vi "Baseband Transmission-Formula.vi"() -> ()   [LabVIEW 2013]
uses:
  <vilib>/Analysis/2dsp.llb/1D Convolution (DBL).vi
  <vilib>/Analysis/2dsp.llb/Decimate (single shot, DBL).vi
  <vilib>/Analysis/2dsp.llb/Upsample (DBL).vi
  <vilib>/Analysis/NI_AALBase.lvlib
  <vilib>/Analysis/NI_AALPro.lvlib
panel:
  in  "alpha":dbl
  in  "Sinc Samples":i32=65
  out "Recovered Bits":i32[](array[numeric])
  in  "stop":bool
  in  "UpSample Factor":i32(slide)=74 scale=1.0..100.0
  out "Symbol":dbl[](array[numeric])
  in  "Bit":i32[](array[numeric])=[0, 0, 0, 1, 0, 1, 1, 1, 0, 0]
  in  "Pulse Shaping Function":enum16{"Sinc ", "Rcosine"}(ring)=enum."Rcosine"
  out "Pulse Shaping":dbl[][](graph)
  out "Baseband":dbl[](graph)
  # "Baseband Transmission"
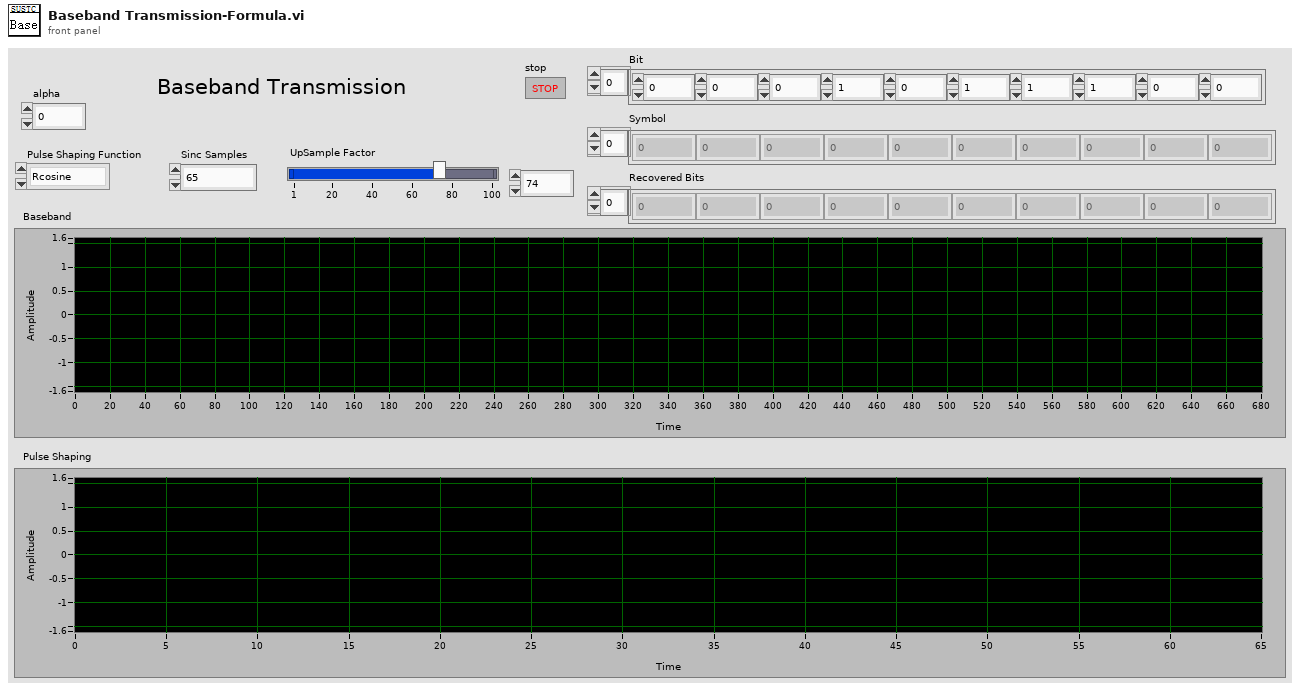
[diagram p1: front panel]
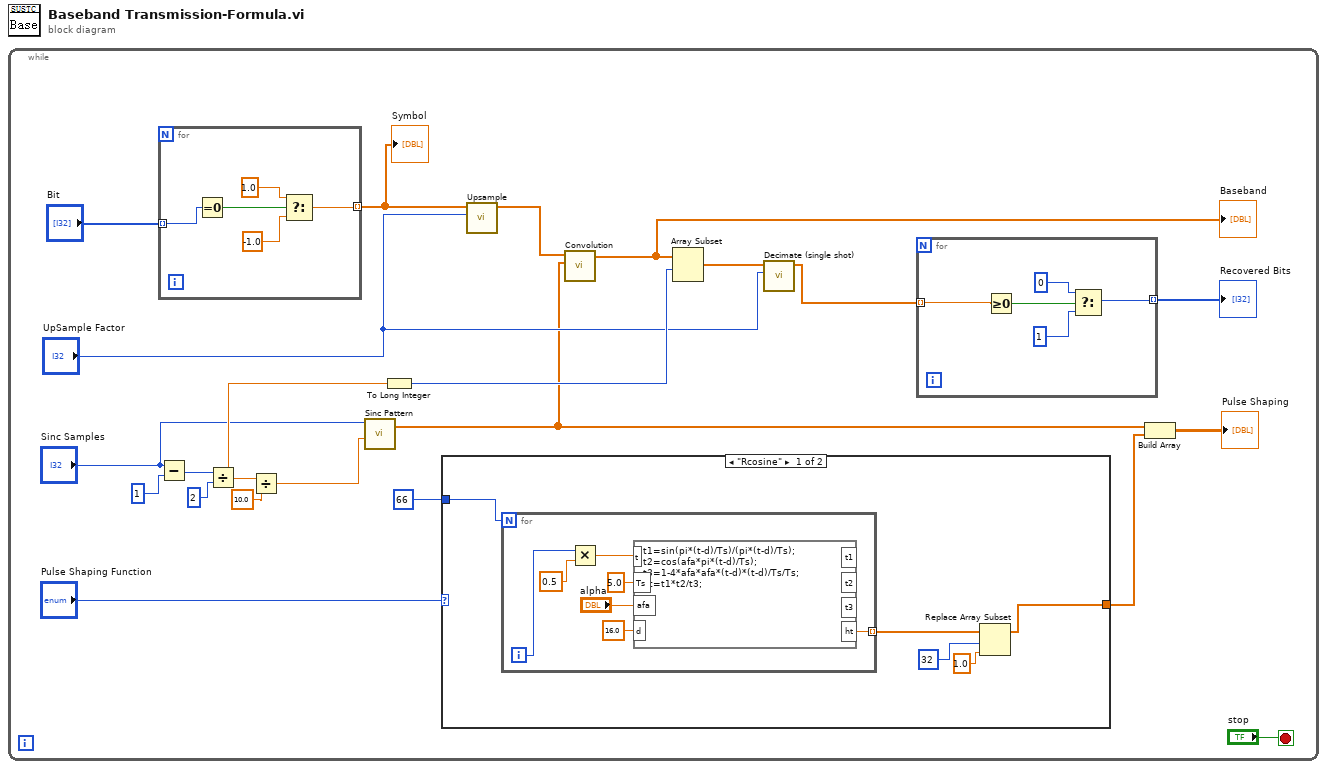
[diagram p0: block diagram]
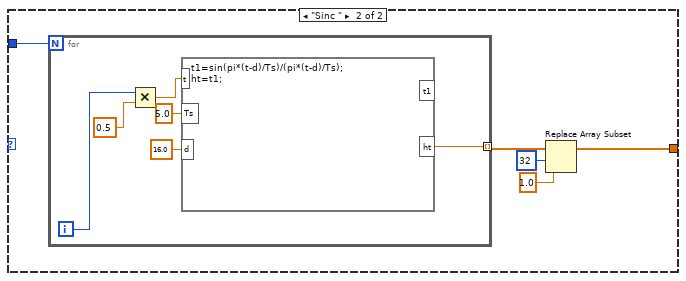
[diagram p2: hidden frame]
diagram:
  n1 = while {
    stop <- "stop" stop-if-true
    n2 = for {
      tunnel: [w52] -> w11 mode=indexing
      tunnel: "Bit" -> [w51] mode=indexing
      n3 = Equal To 0?(x=w51) -> (x = 0?=w55:bool)
      n4 = Select(t=1.0, s=w55, f=-1.0) -> (s? t:f=w52:dbl)
    }
    "Symbol" <- w11
    n5 = Subtract(x="Sinc Samples", y=1) -> (x-y=w19:i32)
    n6 = Divide(x=w19, y=2) -> (x/y=w15:dbl)
    n7 = Divide(x=w15, y=10.0) -> (x/y=w16:dbl)
    n8 = call <vilib>:"Sinc Pattern.vi"("delay"=w16, "samples"="Sinc Samples") -> ("Sinc Pattern"=w2:dbl[])  [unwired: 2 in, 1 out]
    n9 = To Long Integer(number=w15) -> (32bit integer=w7:i32)
    n10 = case shown="\"Rcosine\"" "Pulse Shaping Function" {
      tunnel: 66 -> [w23 w39]
      tunnel: [w24 w37] -> w1
      frame "Rcosine" {
        n11 = for {
          N: w23 -> [_]
          tunnel: [w31] -> w25 mode=indexing
          i -> [w34]
          n12 = Multiply(x=w34, y=0.5) -> (x*y=w32:dbl)
          n13 = formula code="t1=sin(pi*(t-d)/Ts)/(pi*(t-d)/Ts);\nt2=cos(afa*pi*(t-d)/Ts);\nt3=1-4*afa*afa*(t-d)*(t-d)/Ts/Ts;\nht=t1*t2/t3;"("t"=w32, "Ts"=5.0 ("input variable"), "afa"="alpha", "d"=16.0 ("input variable")) -> ("ht"=w31:dbl)  [unwired: 3 out]
        }
        n14 = Replace Array Subset(array=w25, new element=1.0 ("new element/subarray"), index=32) -> (w24:dbl[])
      }
      frame "Sinc " {
        n15 = for {
          N: w39 -> [_]
          tunnel: [w40] -> w38 mode=indexing
          i -> [w45]
          n16 = Multiply(x=w45, y=0.5) -> (x*y=w43:dbl)
          n17 = formula code="t1=sin(pi*(t-d)/Ts)/(pi*(t-d)/Ts);\nht=t1;"("t"=w43, "Ts"=5.0 ("input variable"), "d"=16.0 ("input variable")) -> ("ht"=w40:dbl)  [unwired: 1 out]
        }
        n18 = Replace Array Subset "Replace Array Subset"(array=w38, new element=1.0 ("new element/subarray"), index=32) -> (w37:dbl[])
      }
    }
    n19 = call-poly <vilib>:"Upsample.vi"("upsampling factor"="UpSample Factor", "X"=w11) -> ("Upsampled Array"=w13:dbl[])  [unwired: 8 in, 1 out]
    n20 = call-poly <vilib>:"Convolution.vi"("Y"=w2, "X"=w13) -> ("X * Y"=w8:dbl[])  [unwired: 8 in, 1 out]
    "Baseband" <- w8
    n21 = Array Subset "Array Subset"(array=w8, index=w7) -> (w12:dbl[])  [unwired: 1 in]
    n22 = call-poly <vilib>:"Decimate (single shot).vi"("decimating factor"="UpSample Factor", "X"=w12) -> ("Decimated Array"=w10:dbl[])  [unwired: 8 in, 1 out]
    n23 = for {
      tunnel: w10 -> [w47] mode=indexing
      tunnel: [w48] -> w9 mode=indexing
      n24 = Greater Or Equal To 0?(x=w47) -> (x >= 0?=w46:bool)
      n25 = Select(t=0, s=w46, f=1) -> (s? t:f=w48:i32)
    }
    "Recovered Bits" <- w9
    n26 = Build Array "Build Array"(w2, w1) -> (→"Pulse Shaping":dbl[][])
  }
